vi "ReadbyRef.vi"   [LabVIEW 2010]
doc: "Ce Vi lit la valeur dans le contrôle spécifié par \"Control Ref\""
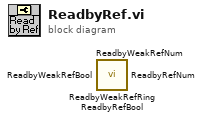
[diagram p0: block diagram]
diagram:
  n1 = call <userlib>:"ReadbyWeakRefRing.vi"() -> ()  [unwired: 10 in, 2 out]
  n2 = call <userlib>:"ReadbyWeakRefNum.vi"() -> ()  [unwired: 10 in, 2 out]
  n3 = call <userlib>:"ReadbyWeakRefBool.vi"() -> ()  [unwired: 10 in, 2 out]
  n4 = call <userlib>:"ReadbyRefNum.vi"() -> ()  [unwired: 10 in, 2 out]
  n5 = call <userlib>:"ReadbyRefBool.vi"() -> ()  [unwired: 10 in, 2 out]
